vi "U3 Counter Read.vi"(8 "error in":errorcluster) -> (0 "error out":errorcluster)   [LabVIEW 2021]
panel:
  out "Counter1":u32
  out "Counter0":u32
  out "Firmware Counter1":u32
  out "Firmware Counter0":u32
  in  "Reset Counter1":bool
  in  "Reset Counter0":bool
  in  "Reset Firmware Counter1":bool
  in  "Reset Firmware Counter0":bool
  # "Reads both firmware counters and both hardware counters.  Must configure first."
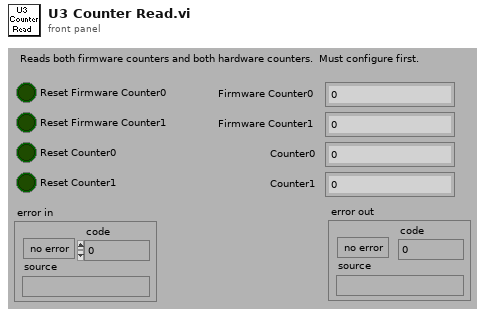
[diagram p1: front panel]
types:
  T1 = cluster{"Open LabJack":bool, "Address":string, "FirstFound":bool}
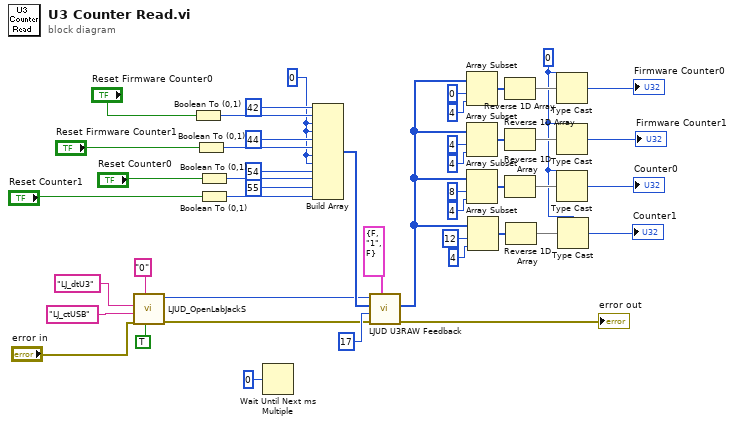
[diagram p0: block diagram]
diagram:
  w10 = u32 0
  w27 = i16 0 ("Input Element")
  n1 = call "LJUD_OpenLabJackS.vi"("FirstFound"=TRUE, "Address"="0", "error in"="error in", "ConnectionType"="LJ_ctUSB", "DeviceType"="LJ_dtU3") -> ("error out"=w29:errorcluster, "Handle"=w28:i32)  [unwired: 4 in, 1 out]
  n2 = Boolean To (0,1)(Boolean="Reset Firmware Counter0") -> (0, 1=w36:i16)
  n3 = Boolean To (0,1)(Boolean="Reset Firmware Counter1") -> (0, 1=w34:i16)
  n4 = Boolean To (0,1)(Boolean="Reset Counter0") -> (0, 1=w32:i16)
  n5 = Boolean To (0,1)(Boolean="Reset Counter1") -> (0, 1=w30:i16)
  n6 = Wait Until Next ms Multiple(millisecond multiple=u32 0) -> ()  [unwired: 1 out]
  n7 = Build Array(u8 42 ("Input Element"), w36, w27, w27, u8 44 ("Input Element"), w34, w27, w27, u8 54 ("Input Element"), w32, u8 55 ("Input Element"), w30) -> (w43:i16[])
  n8 = call "LJUD U3RAW Feedback.vi"("Comm Settings"=T1 {"Open LabJack"=FALSE, "Address"="1", "FirstFound"=FALSE}, "error in (no error)"=w29, "# Data Bytes to Read"=17, "Data"=w43, "Handle In"=w28) -> ("error out"=→"error out":errorcluster, "Data Read"=w9:u8[])  [unwired: 4 in, 1 out]
  n9 = Array Subset(array=w9, index=0 ("Array Index"), length=4 ("Array Length")) -> (w23:u8[])
  n10 = Array Subset(array=w9, index=4 ("Array Index"), length=4 ("Array Length")) -> (w16:u8[])
  n11 = Array Subset(array=w9, index=8 ("Array Index"), length=4 ("Array Length")) -> (w15:u8[])
  n12 = Array Subset(array=w9, index=12 ("Array Index"), length=4 ("Array Length")) -> (w14:u8[])
  n13 = Reverse 1D Array(array=w23) -> (reversed array=w24:u8[])
  n14 = Reverse 1D Array(array=w16) -> (reversed array=w22:u8[])
  n15 = Reverse 1D Array(array=w15) -> (reversed array=w17:u8[])
  n16 = Reverse 1D Array(array=w14) -> (reversed array=w13:u8[])
  n17 = Type Cast(type=w10, x=w24) -> (*(type *) &x=→"Firmware Counter0":u32)
  n18 = Type Cast(type=w10, x=w22) -> (*(type *) &x=→"Firmware Counter1":u32)
  n19 = Type Cast(type=w10, x=w17) -> (*(type *) &x=→"Counter0":u32)
  n20 = Type Cast(type=w10, x=w13) -> (*(type *) &x=→"Counter1":u32)
